vi "3DMathPlot Action String.vi"(11 "Global String":T1 items=["Attribute", "Show/Hide", "Cursor Move", "Zoom", "Mouse Drag", "XY Projection", "YZ Projection", "XZ Projection", "3D Projection", "Active Plot", "Scale"]) -> (3 "String Out":string)   [LabVIEW 2020]
uses:
  <vilib>/Math Plots/3D Math Plots/3D Plot/Action String/3DMathPlot Action String.ctl
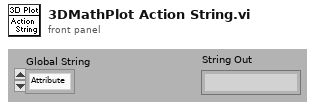
[diagram p1: front panel]
types:
  T1 = typedef "3DMathPlot Action String.ctl" = u16
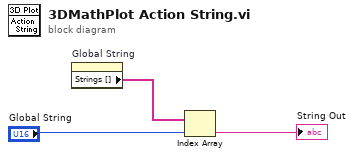
[diagram p0: block diagram]
diagram:
  n1 = property on="Global String" class="Ring (strict)"() -> ("Strings []"=w3:string[])  [unwired: 2 in, 2 out]
  n2 = Index Array(array=w3, index="Global String") -> (element=→"String Out":string)
